vi "gugudan Client.vi"() -> ()   [LabVIEW 2014]
uses:
  <vilib>/Utility/sysdir.llb/System Directory Type.ctl
panel:
  out "email 2":string
  out "ip address":string=" ip address\r\n   서브넷 마스크 . . . . . . . : 255.255.255.0\r\n   기본 게이트웨이 . . . . . . : 192.168.0.1\r\n\r\n터널 어댑터 isatap.{E2E91750-802C-47E4-94E7-F6C5BD44A78B}:\r\n\r\n   미디어 상태 . . . . . . . . : 미디어 연결 끊김\r\n   연결별 DNS 접미사. . . . : \r\n\r\n터널 어댑터 로컬 영역 연결* 2:\r\n\r\n   연결별 DNS 접미사. . . . : \r\n   IPv6 주소 . . . . . . . . . : 2001:0:682f:9980:3c40:17a9:3f57:fff6\r\n   링크-로컬 IPv6 주소 . . . . : fe80::3c40:17a9:3f57:fff6%12\r\n   기본 게이트웨이 . . . . . . : ::\r\n"
  in  "제한해제":bool
  out "TIME":string="현재날자,시간"
  out "배열":string[][](array[string])
  out "email":string
  out "연결된 문자열":string
  out "abs(x)":i32
  out "문자열":string
  out "스페이스바3 2":string
  out "A  2":string
  out "D  2":string
  out "W 2":string
  out "W":string
  out "D":string
  out "A":string
  out "1":string
  out "2":string
  out "3":string
  out "스페이스바3":string
  out "key의숫자값":i16[](array[numeric])
  # "서비스를 이용해 주셔 감사합니다."
  # "서비스 종료를 위해서는 관리자 암호를 입력 해야 종료가 가능합니다."
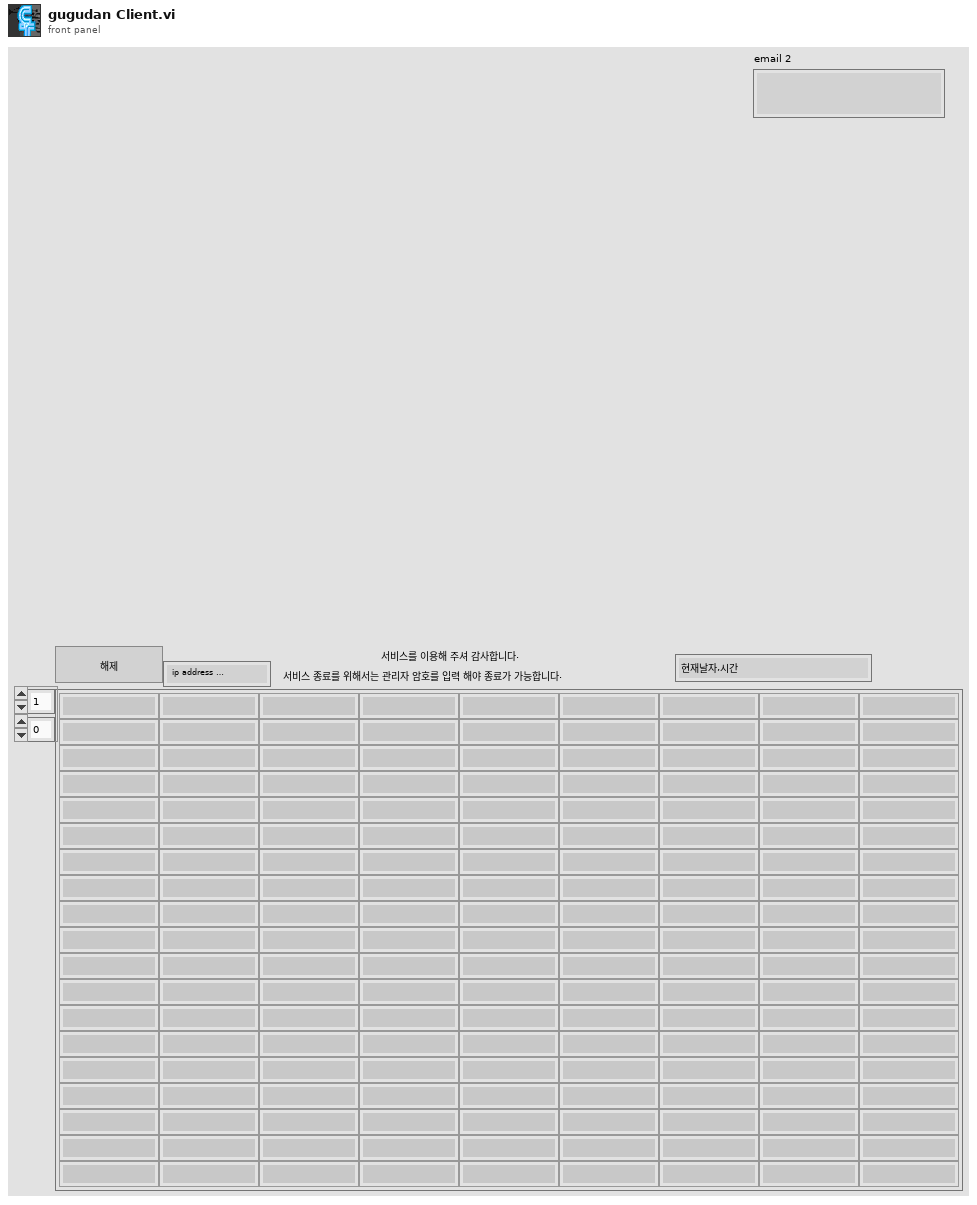
[diagram p1: front panel]
types:
  T1 = enum16{"open", "replace", "create", "open or create", "replace or create", "replace or create with confirmation"}
  T2 = typedef "System Directory Type.ctl" = i32
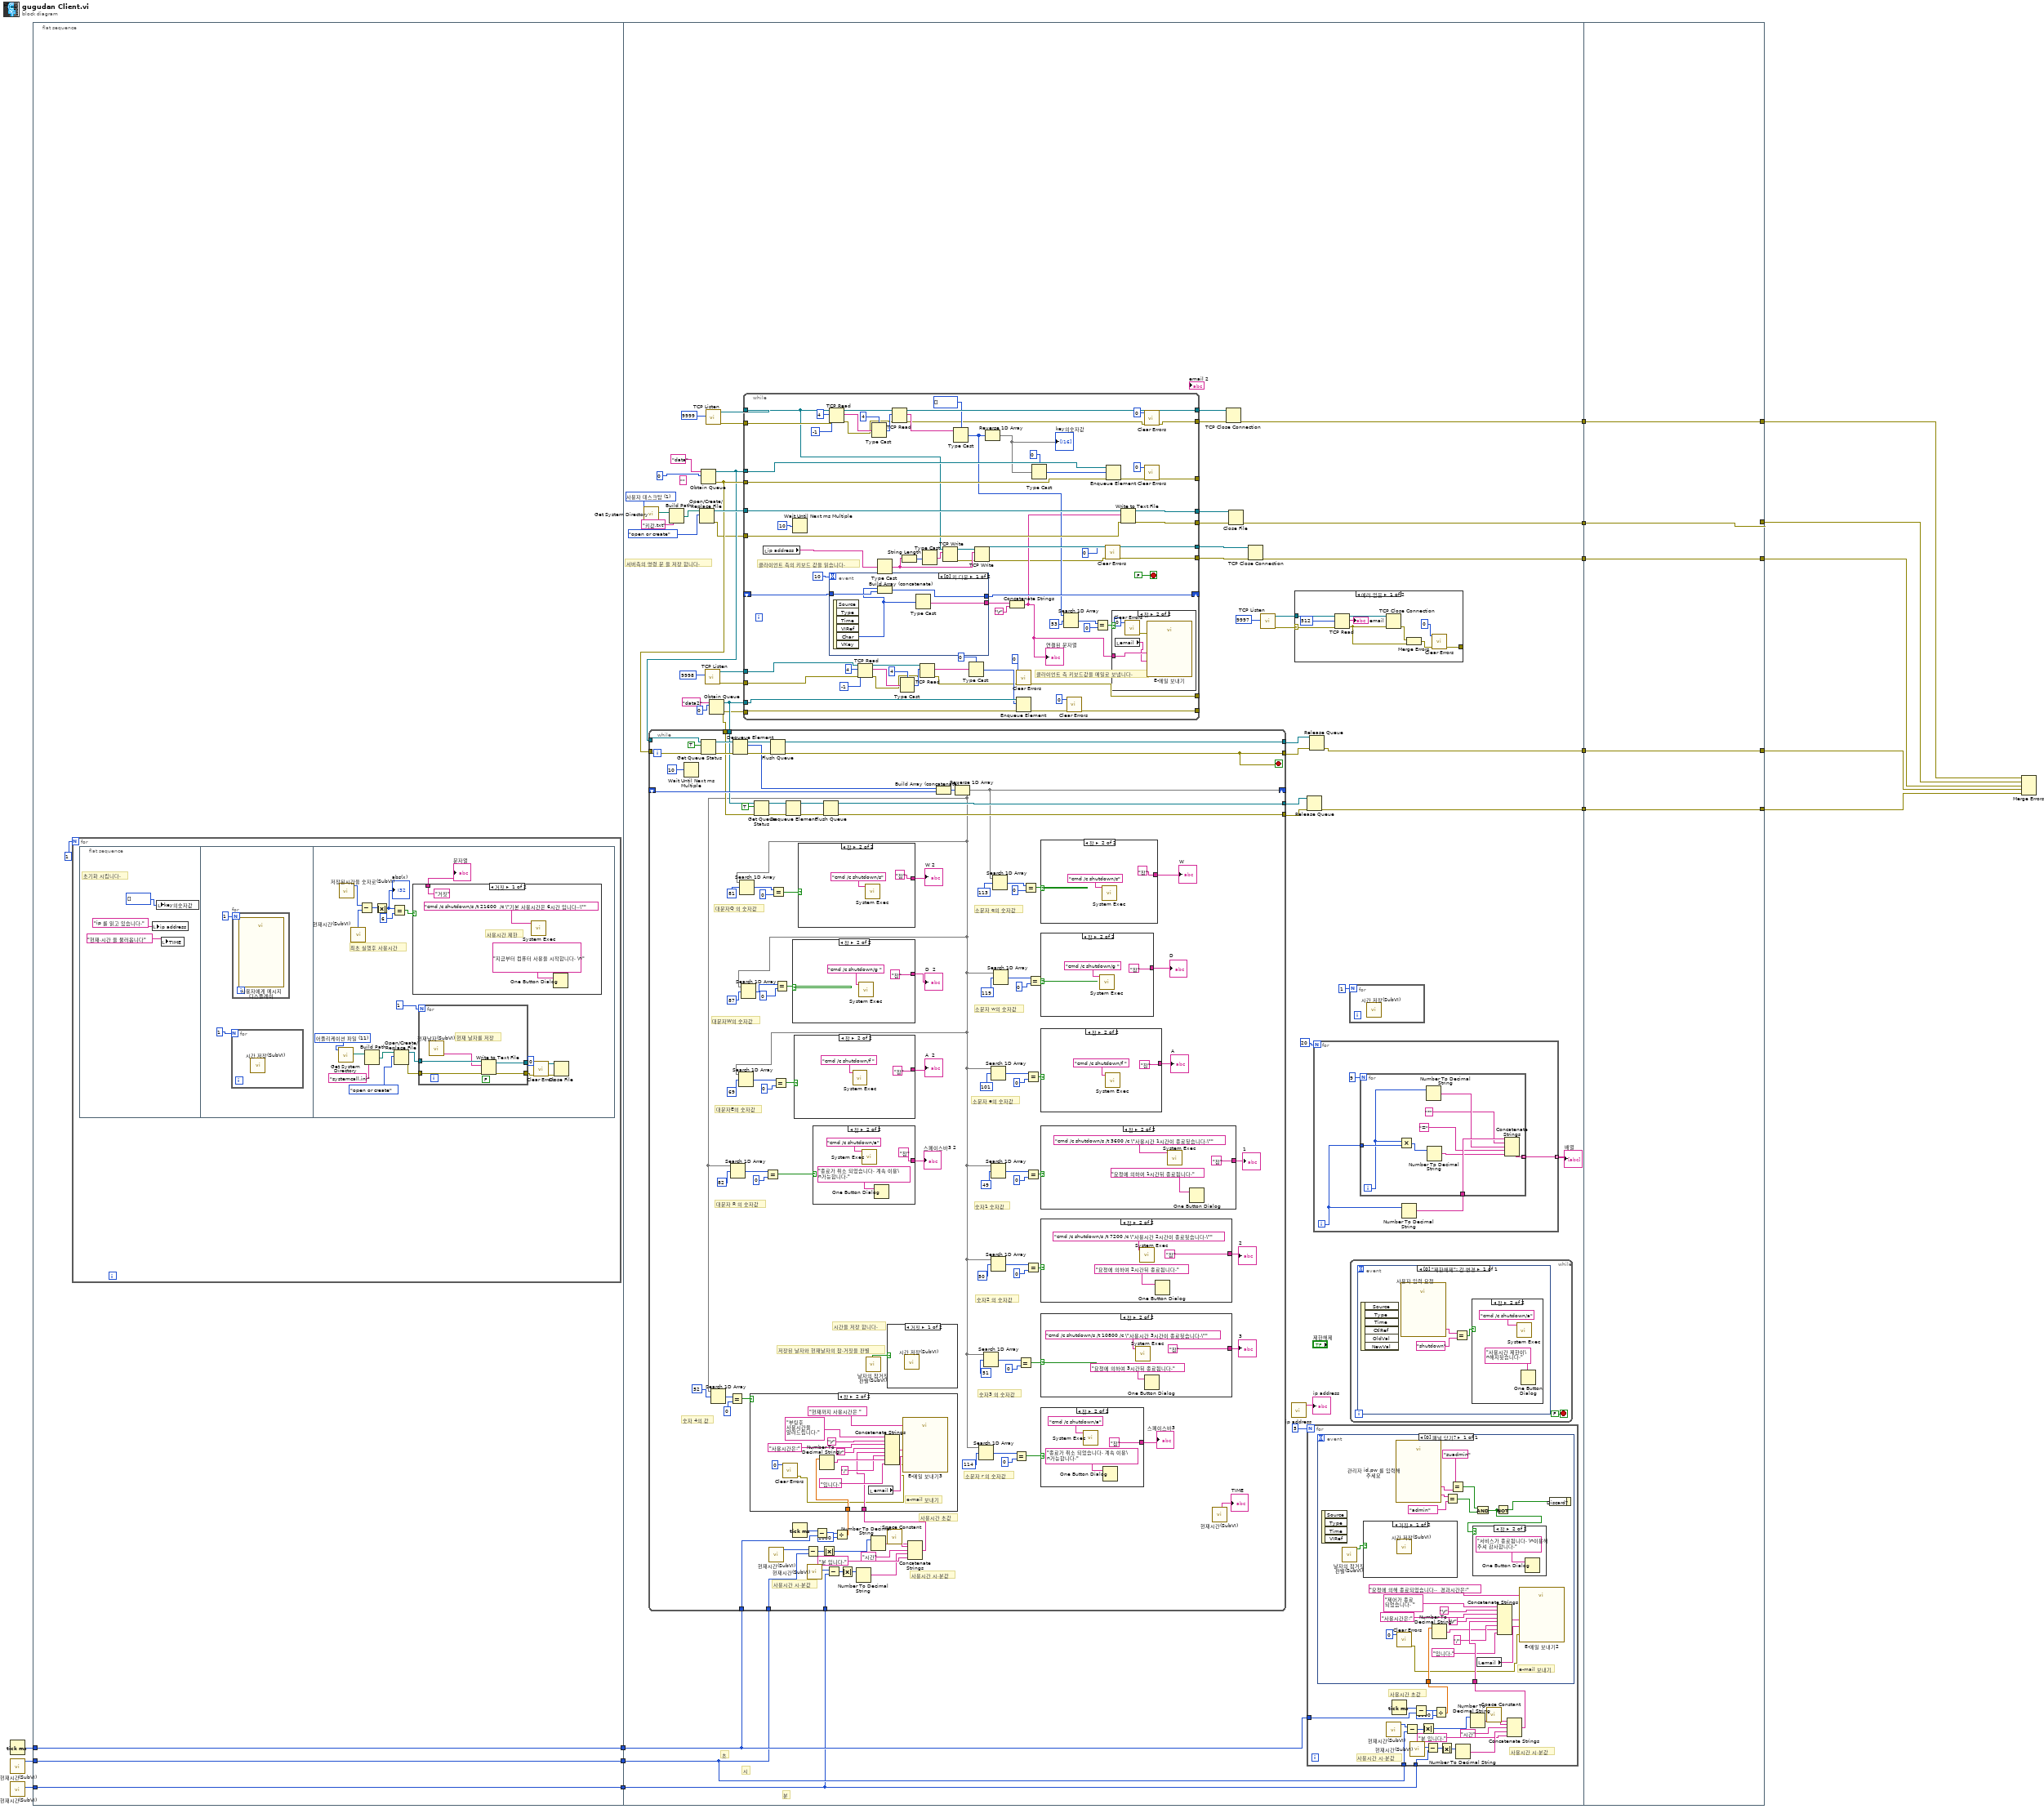
[diagram p0: block diagram]
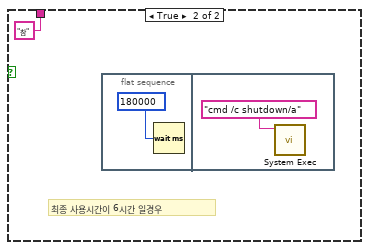
[diagram p2: hidden frame]
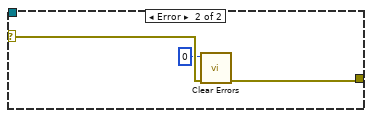
[diagram p4: hidden frame]
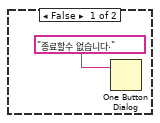
[diagram p6: hidden frame]
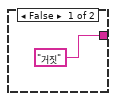
[diagram p9: hidden frame]
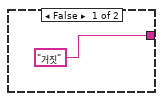
[diagram p10: hidden frame]
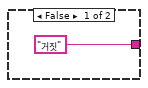
[diagram p11: hidden frame]
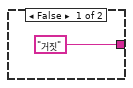
[diagram p12: hidden frame]
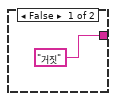
[diagram p13: hidden frame]
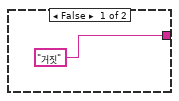
[diagram p14: hidden frame]
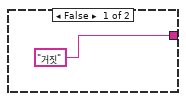
[diagram p15: hidden frame]
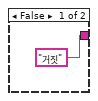
[diagram p16: hidden frame]
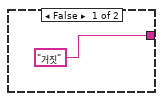
[diagram p17: hidden frame]
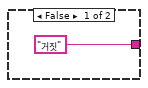
[diagram p18: hidden frame]
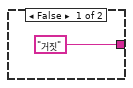
[diagram p19: hidden frame]
diagram:
  n1 = Tick Count (ms)() -> (millisecond timer value=w5:u32)
  n2 = call "현재시간(SubVI).vi"() -> ("시"=w4:i32)  [unwired: 3 in, 8 out]
  n3 = call "현재시간(SubVI).vi"() -> ("분"=w3:i32)  [unwired: 3 in, 8 out]
  n4 = flat-sequence {
    tunnel: [w19] -> w6
    tunnel: w5 -> [w19]
    tunnel: w4 -> [w18]
    tunnel: w3 -> [w17]
    tunnel: [w18] -> w2
    tunnel: [w17] -> w1
    tunnel: [w76] -> w16
    tunnel: [w67] -> w15
    tunnel: [w75] -> w14
    tunnel: [w74] -> w13
    tunnel: [w73] -> w12
    tunnel: w6 -> [w65]
    tunnel: w2 -> [w64]
    tunnel: w1 -> [w63]
    tunnel: w16 -> [w417]
    tunnel: w15 -> [w416]
    tunnel: w14 -> [w415]
    tunnel: w13 -> [w414]
    tunnel: w12 -> [w413]
    tunnel: [w417] -> w9
    tunnel: [w416] -> w8
    tunnel: [w415] -> w7
    tunnel: [w414] -> w10
    tunnel: [w413] -> w11
    frame #0 {
      n5 = for {
        N: 1 -> [_]
        n6 = flat-sequence {
          frame #0 {
            # "초기화 시킵니다."
            n7 = local write "ip address"("ip 를 읽고 있습니다.") -> ()
            n8 = local write "key의숫자값"(i16[] []) -> ()
            n9 = local write "TIME"("현재,시간 을 불러옵니다") -> ()
          }
          frame #1 {
            n10 = for {
              N: 1 -> [_]
              n11 = call "시간 저장(SubVI).vi"() -> ()  [unwired: 12 in]
            }
            n12 = for {
              N: 1 -> [_]
              n13 = call "사용자에게 메시지 디스플레이"() -> ()  [unwired: 10 in, 2 out]
            }
          }
          frame #2 {
            w28 = T2 11 items=["사용자 홈"=0, "사용자 데스크탑"=1, "사용자 문서"=2, "사용자 어플리케이션 데이터"=3, "사용자 환경"=4, "사용자 임시"=5, "퍼블릭 문서"=6, "퍼블릭 어플리케이션 데이터"=7, "퍼블릭 환경"=8, "퍼블릭 캐시"=13, "시스템 코어 라이브러리"=9, "시스템 설치된 라이브러리"=10, "어플리케이션 파일"=11, "부팅 볼륨 루트"=12] ("system directory type")
            # "최초 실행후 사용시간"
            n14 = call <vilib>:"Get System Directory.vi"("system directory type"=w28) -> ("system directory"=w33:path)  [unwired: 10 in]
            n15 = call "저장된시간을 숫자로(SubVI).vi"() -> ("저장된 문자를 숫자로"=w38:i32)  [unwired: 11 in]
            n16 = call "현재시간(SubVI).vi"() -> ("시"=w39:i32)  [unwired: 3 in, 8 out]
            n17 = Subtract(x=w38, y=w39) -> (x-y=w40:i32)
            n18 = Build Path(base path=w33, name or relative path="systemcall.ini" ("이름 또는 상대 경로")) -> (appended path=w31:path)
            n19 = Absolute Value(x=w40) -> (abs(x)=w42:i32)
            "abs(x)" <- w42
            n20 = Equal?(x=w42, y=6) -> (x = y?=w44:bool)
            n21 = Open/Create/Replace File(file path (use dialog)=w31, operation (0:open)=T1."open or create" ("동작(0:open)")) -> (refnum out=w29:refnum<file>, error out=w30:errorcluster)  [unwired: 4 in, 1 out]
            n22 = case shown="거짓" w44 {
              tunnel: ["거짓" "참"] -> w41
              frame False {
                # "사용시간 제한"
                n23 = call <vilib>:"System Exec.vi"("command line"="cmd /c shutdown/s /t 21600  /c \"기본 사용시간은 6시간 입니다..\"" ("standard input")) -> ()  [unwired: 7 in, 4 out]
                n24 = One Button Dialog(message="지금부터 컴퓨터 사용을 시작합니다. \n" ("메시지")) -> ()  [unwired: 1 in, 1 out]
              }
              frame True {
                # "최종 사용시간이 6시간 일경우"
                n25 = flat-sequence {
                  frame #0 {
                    n26 = Wait (ms)(milliseconds to wait=u32 180000 ("대기 시간(ms)")) -> ()  [unwired: 1 out]
                  }
                  frame #1 {
                    n27 = call <vilib>:"System Exec.vi"("command line"="cmd /c shutdown/a" ("standard input")) -> ()  [unwired: 7 in, 4 out]
                  }
                }
              }
            }
            "문자열" <- w41
            n28 = for {
              N: 1 -> [_]
              tunnel: w30 -> [w49]
              tunnel: [w48] -> w35
              tunnel: [w47] -> w34
              tunnel: w29 -> [w46]
              (unwired) FALSE
              # "현재 날자를 저장"
              n29 = call "현재날자(SubVI).vi"() -> ("월,일 을 문자열로"=w45:string)  [unwired: 5 in, 6 out]
              n30 = Write to Text File(file (use dialog)=w46, text=w45, error in=w49) -> (refnum out=w47:refnum<file>, error out=w48:errorcluster)  [unwired: 1 in, 1 out]
            }
            n31 = call <vilib>:"Clear Errors.vi"("error in (no error)"=w35, "specific error code to clear (0: all)"=0) -> ("error out"=w36:errorcluster)  [unwired: 4 in, 1 out]
            n32 = Close File(refnum=w34, error in=w36) -> ()  [unwired: 2 out]
          }
        }
      }
    }
    frame #1 {
      (unwired) ""
      w97 = T2 1 items=["사용자 홈"=0, "사용자 데스크탑"=1, "사용자 문서"=2, "사용자 어플리케이션 데이터"=3, "사용자 환경"=4, "사용자 임시"=5, "퍼블릭 문서"=6, "퍼블릭 어플리케이션 데이터"=7, "퍼블릭 환경"=8, "퍼블릭 캐시"=13, "시스템 코어 라이브러리"=9, "시스템 설치된 라이브러리"=10, "어플리케이션 파일"=11, "부팅 볼륨 루트"=12] ("system directory type")
      # "서버측의 명령 문 을 저장 합니다."
      # "초"
      # "분"
      # "시"
      n33 = call <vilib>:"Get System Directory.vi"("system directory type"=w97) -> ("system directory"=w96:path)  [unwired: 10 in]
      n34 = Build Path(base path=w96, name or relative path="키값.txt" ("이름 또는 상대 경로")) -> (appended path=w93:path)
      n35 = Open/Create/Replace File(file path (use dialog)=w93, operation (0:open)=T1."open or create" ("동작(0:open)")) -> (refnum out=w92:refnum<file>, error out=w71:errorcluster)  [unwired: 4 in, 1 out]
      n36 = Obtain Queue(name (unnamed)="data" ("이름(이름없음)"), element data type=i16 0) -> (queue out=w86:refnum<queue>, error out=w87:errorcluster)  [unwired: 3 in, 1 out]
      n37 = call <vilib>:"TCP Listen.vi"("port"=u16 9998) -> ("error out"=w83:errorcluster, "connection ID"=w84:refnum<k5>)  [unwired: 6 in, 3 out]
      n38 = call <vilib>:"TCP Listen.vi"("port"=u16 9999) -> ("error out"=w68:errorcluster, "connection ID"=w100:refnum<k5>)  [unwired: 6 in, 3 out]
      n39 = Obtain Queue(name (unnamed)="data2" ("이름(이름없음)"), element data type=i16 0) -> (queue out=w78:refnum<queue>, error out=w77:errorcluster)  [unwired: 3 in, 1 out]
      n40 = while {
        shift-right: [w180] -> _
        shift-left: _ -> [w245]
        tunnel: [w238] -> w89
        tunnel: [w237] -> w88
        tunnel: w86 -> [w244]
        tunnel: w87 -> [w243]
        tunnel: [w228] -> w80
        tunnel: [w227] -> w79
        tunnel: w78 -> [w206]
        tunnel: w77 -> [w205]
        tunnel: w65 -> [w185]
        tunnel: w64 -> [w184]
        tunnel: w63 -> [w183]
        stop <- w237 stop-if-true
        # "숫자 4의 값"
        # "저장된 날자와 현재날자의 참,거짓을 판별"
        # "시간을 저장 합니다."
        # "사용시간 시,분값"
        # "사용시간 시,분값"
        # "사용시간 초값"
        # "대문자 R 의 숫자값"
        # "대문자Q 의 숫자값"
        # "대문자W의 숫자값"
        # "대문자E의 숫자값"
        # "소문자 r 의 숫자값"
        # "숫자3 의 숫자값"
        # "소문자 q의 숫자값"
        # "소문자 w의 숫자값"
        # "소문자 e의 숫자값"
        # "숫자1 숫자값"
        # "숫자2 의 숫자값"
        n41 = Wait Until Next ms Multiple(millisecond multiple=u32 10) -> ()  [unwired: 1 out]
        n42 = Get Queue Status(queue=w244, return elements? (F)=TRUE ("원소 반환? (거짓)"), error in (no error)=w243) -> (queue out=w242:refnum<queue>, error out=w241:errorcluster)  [unwired: 6 out]
        n43 = Dequeue Element(queue=w242, error in (no error)=w241) -> (queue out=w239:refnum<queue>, element=w236:i16, error out=w240:errorcluster)  [unwired: 1 in, 1 out]
        n44 = Get Queue Status(queue=w206, return elements? (F)=TRUE ("원소 반환? (거짓)"), error in (no error)=w205) -> (queue out=w232:refnum<queue>, error out=w231:errorcluster)  [unwired: 6 out]
        n45 = call "현재시간(SubVI).vi"() -> ("시"=w187:i32)  [unwired: 3 in, 8 out]
        n46 = Flush Queue(queue=w239, error in (no error)=w240) -> (queue out=w238:refnum<queue>, error out=w237:errorcluster)  [unwired: 1 out]
        n47 = Dequeue Element(queue=w232, error in (no error)=w231) -> (queue out=w229:refnum<queue>, error out=w230:errorcluster)  [unwired: 1 in, 2 out]
        n48 = Tick Count (ms)() -> (millisecond timer value=w186:u32)
        n49 = Subtract(x=w187, y=w184) -> (x-y=w189:i32)
        n50 = call "현재시간(SubVI).vi"() -> ("분"=w188:i32)  [unwired: 3 in, 8 out]
        n51 = Subtract(x=w186, y=w185) -> (x-y=w198:u32)
        n52 = Absolute Value(x=w189) -> (abs(x)=w191:i32)
        n53 = Flush Queue(queue=w229, error in (no error)=w230) -> (queue out=w227:refnum<queue>, error out=w228:errorcluster)  [unwired: 1 out]
        n54 = Subtract(x=w188, y=w183) -> (x-y=w190:i32)
        n55 = Divide(x=w198, y=u32 1000) -> (x/y=w182:dbl)
        n56 = Absolute Value(x=w190) -> (abs(x)=w192:i32)
        n57 = Number To Decimal String(number=w192) -> (decimal integer string=w194:string)  [unwired: 1 in]
        n58 = call "날자의 참거짓 판별(SubVI).vi"() -> ("불리언"=w204:bool)  [unwired: 9 in, 2 out]
        n59 = Number To Decimal String(number=w191) -> (decimal integer string=w196:string)  [unwired: 1 in]
        n60 = call <vilib>:"Space Constant.vi"() -> ("String"=w197:string)
        n61 = case shown="거짓" w204 {
          frame False {
            n62 = call "시간 저장(SubVI).vi"() -> ()  [unwired: 12 in]
          }
          frame True {
          }
        }
        n63 = Concatenate Strings(w196, w197, "시간", w194, "분 입니다.") -> (w181:string)
        n64 = Build Array (concatenate)(w236, w245) -> (w234:i16[])
        n65 = Reverse 1D Array(array=w234) -> (reversed array=w180:i16[])
        n66 = Search 1D Array(1D array=w180, element=i16 52 ("원소")) -> (index of element=w202:i32)  [unwired: 1 in]
        n67 = Equal?(x=w202, y=0) -> (x = y?=w200:bool)
        n68 = Search 1D Array(1D array=w180, element=i16 82 ("원소")) -> (index of element=w209:i32)  [unwired: 1 in]
        n69 = Search 1D Array(1D array=w180, element=i16 69 ("원소")) -> (index of element=w214:i32)  [unwired: 1 in]
        n70 = Search 1D Array(1D array=w180, element=i16 81 ("원소")) -> (index of element=w224:i32)  [unwired: 1 in]
        n71 = Search 1D Array(1D array=w180, element=i16 87 ("원소")) -> (index of element=w222:i32)  [unwired: 1 in]
        n72 = case shown="참" w200 {
          tunnel: w182 -> [_ w286]
          tunnel: w181 -> [_ w285]
          frame False {
          }
          frame True {
            # "e-mail 보내기"
            n73 = call <vilib>:"Clear Errors.vi"("specific error code to clear (0: all)"=0) -> ("error out"=w282:errorcluster)  [unwired: 5 in, 1 out]
            n74 = Number To Decimal String(number=w286) -> (decimal integer string=w294:string)  [unwired: 1 in]
            n75 = local read "email"() -> (w284:string)
            n76 = Concatenate Strings("부팅후 사용시간을 알려드립니다." ("문자열"), "\r", "사용시간은:", "\r", w285, "/", w294, "입니다.") -> (w291:string)
            n77 = call "E-메일 보내기3"("error in"=w282, "Message"=w291, "Subject"="현재까지 사용시간은 ", "Recipients"=w284) -> ()  [unwired: 7 in, 1 out]
          }
        }
        n78 = Equal?(x=w209, y=0) -> (x = y?=w211:bool)
        n79 = Equal?(x=w224, y=0) -> (x = y?=w221:bool)
        n80 = Equal?(x=w214, y=0) -> (x = y?=w216:bool)
        n81 = Equal?(x=w222, y=0) -> (x = y?=w219:bool)
        n82 = case shown="참" w219 {
          tunnel: ["거짓" "참"] -> w220
          frame False {
          }
          frame True {
            n83 = call <vilib>:"System Exec.vi"("command line"="cmd /c shutdown/g " ("standard input")) -> ()  [unwired: 7 in, 4 out]
          }
        }
        "D  2" <- w220
        n84 = case shown="참" w216 {
          tunnel: ["거짓" "참"] -> w215
          frame False {
          }
          frame True {
            n85 = call <vilib>:"System Exec.vi"("command line"="cmd /c shutdown/f " ("standard input")) -> ()  [unwired: 7 in, 4 out]
          }
        }
        "A  2" <- w215
        n86 = case shown="참" w221 {
          tunnel: ["거짓" "참"] -> w226
          frame False {
          }
          frame True {
            n87 = call <vilib>:"System Exec.vi"("command line"="cmd /c shutdown/s" ("standard input")) -> ()  [unwired: 7 in, 4 out]
          }
        }
        "W 2" <- w226
        n88 = case shown="참" w211 {
          tunnel: ["거짓" "참"] -> w207
          frame False {
          }
          frame True {
            n89 = call <vilib>:"System Exec.vi"("command line"="cmd /c shutdown/a" ("standard input")) -> ()  [unwired: 7 in, 4 out]
            n90 = One Button Dialog(message="종료가 취소 되었습니다. 계속 이용\n가능합니다." ("메시지")) -> ()  [unwired: 1 in, 1 out]
          }
        }
        "스페이스바3 2" <- w207
        n91 = Search 1D Array(1D array=w180, element=i16 114 ("원소")) -> (index of element=w250:i32)  [unwired: 1 in]
        n92 = Search 1D Array(1D array=w180, element=i16 51 ("원소")) -> (index of element=w255:i32)  [unwired: 1 in]
        n93 = Search 1D Array(1D array=w180, element=i16 101 ("원소")) -> (index of element=w269:i32)  [unwired: 1 in]
        n94 = Search 1D Array(1D array=w180, element=i16 49 ("원소")) -> (index of element=w268:i32)  [unwired: 1 in]
        n95 = Search 1D Array(1D array=w180, element=i16 50 ("원소")) -> (index of element=w261:i32)  [unwired: 1 in]
        n96 = Search 1D Array(1D array=w180, element=i16 113 ("원소")) -> (index of element=w279:i32)  [unwired: 1 in]
        n97 = Search 1D Array(1D array=w180, element=i16 119 ("원소")) -> (index of element=w277:i32)  [unwired: 1 in]
        n98 = Equal?(x=w250, y=0) -> (x = y?=w252:bool)
        n99 = Equal?(x=w255, y=0) -> (x = y?=w253:bool)
        n100 = Equal?(x=w279, y=0) -> (x = y?=w276:bool)
        n101 = Equal?(x=w269, y=0) -> (x = y?=w271:bool)
        n102 = Equal?(x=w268, y=0) -> (x = y?=w266:bool)
        n103 = Equal?(x=w261, y=0) -> (x = y?=w263:bool)
        n104 = Equal?(x=w277, y=0) -> (x = y?=w274:bool)
        n105 = case shown="참" w276 {
          tunnel: ["거짓" "참"] -> w281
          frame False {
          }
          frame True {
            n106 = call <vilib>:"System Exec.vi"("command line"="cmd /c shutdown/s" ("standard input")) -> ()  [unwired: 7 in, 4 out]
          }
        }
        "W" <- w281
        n107 = case shown="참" w274 {
          tunnel: ["거짓" "참"] -> w275
          frame False {
          }
          frame True {
            n108 = call <vilib>:"System Exec.vi"("command line"="cmd /c shutdown/g " ("standard input")) -> ()  [unwired: 7 in, 4 out]
          }
        }
        "D" <- w275
        n109 = case shown="참" w271 {
          tunnel: ["거짓" "참"] -> w270
          frame False {
          }
          frame True {
            n110 = call <vilib>:"System Exec.vi"("command line"="cmd /c shutdown/f " ("standard input")) -> ()  [unwired: 7 in, 4 out]
          }
        }
        "A" <- w270
        n111 = case shown="참" w266 {
          tunnel: ["거짓" "참"] -> w267
          frame False {
          }
          frame True {
            n112 = call <vilib>:"System Exec.vi"("command line"="cmd /c shutdown/s /t 3600 /c \"사용시간 1시간이 종료됫습니다.\"" ("standard input")) -> ()  [unwired: 7 in, 4 out]
            n113 = One Button Dialog(message="요청에 의하여 1시간뒤 종료됩니다." ("메시지")) -> ()  [unwired: 1 in, 1 out]
          }
        }
        "1" <- w267
        n114 = case shown="참" w263 {
          tunnel: ["거짓" "참"] -> w262
          frame False {
          }
          frame True {
            n115 = call <vilib>:"System Exec.vi"("command line"="cmd /c shutdown/s /t 7200 /c \"사용시간 2시간이 종료됫습니다.\"" ("standard input")) -> ()  [unwired: 7 in, 4 out]
            n116 = One Button Dialog(message="요청에 의하여 2시간뒤 종료됩니다." ("메시지")) -> ()  [unwired: 1 in, 1 out]
          }
        }
        "2" <- w262
        n117 = case shown="참" w253 {
          tunnel: ["거짓" "참"] -> w235
          frame False {
          }
          frame True {
            n118 = call <vilib>:"System Exec.vi"("command line"="cmd /c shutdown/s /t 10800 /c \"사용시간 3시간이 종료됫습니다.\"" ("standard input")) -> ()  [unwired: 7 in, 4 out]
            n119 = One Button Dialog(message="요청에 의하여 3시간뒤 종료됩니다." ("메시지")) -> ()  [unwired: 1 in, 1 out]
          }
        }
        "3" <- w235
        n120 = case shown="참" w252 {
          tunnel: ["거짓" "참"] -> w248
          frame False {
          }
          frame True {
            n121 = call <vilib>:"System Exec.vi"("command line"="cmd /c shutdown/a" ("standard input")) -> ()  [unwired: 7 in, 4 out]
            n122 = One Button Dialog(message="종료가 취소 되었습니다. 계속 이용\n가능합니다." ("메시지")) -> ()  [unwired: 1 in, 1 out]
          }
        }
        "스페이스바3" <- w248
        n123 = call "현재시간(SubVI).vi"() -> ("날짜/시간 문자열"=→"TIME":string)  [unwired: 3 in, 8 out]
      }
      n124 = while {
        tunnel: w100 -> [w334]
        tunnel: [w403] -> w101
        tunnel: [w396] -> w99
        tunnel: w92 -> [w389]
        tunnel: [w390] -> w98
        tunnel: w86 -> [w388]
        tunnel: w87 -> [w387]
        shift-right: [w379] -> _
        shift-left: _ -> [w380]
        tunnel: w84 -> [w335]
        tunnel: w83 -> [w371]
        tunnel: w78 -> [w366]
        tunnel: w77 -> [w367]
        tunnel: [w339] -> w72
        tunnel: w71 -> [w363]
        tunnel: [w362] -> w70
        tunnel: [w351] -> w69
        tunnel: w68 -> [w360]
        tunnel: [w348] -> _
        tunnel: [w344] -> _
        tunnel: [w341] -> _
        stop <- FALSE stop-if-true
        # "클라이언트 측 키보드값을 메일로 보냅니다."
        # "클라이언트 측의 키보드 값을 읽습니다."
        n125 = local read "ip address"() -> (w336:string)
        n126 = Wait Until Next ms Multiple(millisecond multiple=u32 10) -> ()  [unwired: 1 out]
        n127 = TCP Read(connection ID=w334, bytes to read=4, error in (no error)=w360, 9:-1 ("타임아웃 ms (25000)")) -> (connection ID out=w393:refnum<k5>, data out=w395:string, error out=w361:errorcluster)  [unwired: 1 in]
        n128 = event shown="[0] 키 다운" {
          selector: _ -> [_ _]
          dyn-events: _ -> [_ _]
          timeout: 10 -> [_ _]
          tunnel: [w410 w412] -> w379
          tunnel: w380 -> [w411 w412]
          tunnel: [w408 _] -> w359
          event Key Down {
            n129 = event-data() -> ("Char"=w409:i16)  [unwired: 1 in, 5 out]
            n130 = Build Array (concatenate)(w409, w411) -> (w410:i16[])
            n131 = Type Cast(x=w409) -> (*(type *) &x=w408:string)  [unwired: 1 in]
          }
          event Timeout {
            n132 = event-data() -> ()  [unwired: 1 in, 3 out]
          }
        }
        n133 = TCP Read(connection ID=w335, bytes to read=4, error in (no error)=w371, 9:-1 ("타임아웃 ms (25000)")) -> (connection ID out=w374:refnum<k5>, data out=w372:string, error out=w370:errorcluster)  [unwired: 1 in]
        n134 = Type Cast(type=4 ("bytes to read"), x=w395) -> (*(type *) &x=w385:i32)
        n135 = Type Cast(x=w336) -> (*(type *) &x=w397:string)  [unwired: 1 in]
        n136 = TCP Read(connection ID=w393, bytes to read=w385, error in (no error)=w361) -> (connection ID out=w403:refnum<k5>, data out=w386:string, error out=w350:errorcluster)  [unwired: 2 in]
        n137 = Type Cast(type=4 ("bytes to read"), x=w372) -> (*(type *) &x=w377:i32)
        n138 = String Length(string=w397) -> (length=w398:i32)
        n139 = TCP Read(connection ID=w374, bytes to read=w377, error in (no error)=w370) -> (data out=w369:string, error out=w342:errorcluster)  [unwired: 2 in, 1 out]
        n140 = Type Cast(x=w398) -> (*(type *) &x=w399:string)  [unwired: 1 in]
        n141 = TCP Write(connection ID=w334, data in=w399) -> (connection ID out=w400:refnum<k5>, error out=w364:errorcluster)  [unwired: 2 in, 1 out]
        n142 = Type Cast(type=i16[] [], x=w386) -> (*(type *) &x=w354:i16[])
        n143 = Type Cast(type=i16 0, x=w369) -> (*(type *) &x=w365:i16)
        n144 = TCP Write(connection ID=w400, data in=w397, error in (no error)=w364) -> (connection ID out=w396:refnum<k5>, error out=w338:errorcluster)  [unwired: 1 in, 1 out]
        n145 = Reverse 1D Array(array=w354) -> (reversed array=w381:i16[])
        "key의숫자값" <- w381
        n146 = Concatenate Strings(w359, "\r") -> (w352:string)
        "연결된 문자열" <- w352
        n147 = Enqueue Element(queue=w366, element=w365, error in (no error)=w367) -> (error out=w345:errorcluster)  [unwired: 1 in, 2 out]
        n148 = call <vilib>:"Clear Errors.vi"("error in (no error)"=w342, "specific error code to clear (0: all)"=0) -> ("error out"=w341:errorcluster)  [unwired: 4 in, 1 out]
        n149 = Type Cast(type=i16 0, x=w381) -> (*(type *) &x=w383:i16)
        n150 = Search 1D Array(1D array=w354, element=i16 53 ("원소")) -> (index of element=w357:i32)  [unwired: 1 in]
        n151 = call <vilib>:"Clear Errors.vi"("error in (no error)"=w345, "specific error code to clear (0: all)"=0) -> ("error out"=w344:errorcluster)  [unwired: 4 in, 1 out]
        n152 = Equal?(x=w357, y=0) -> (x = y?=w353:bool)
        n153 = call <vilib>:"Clear Errors.vi"("error in (no error)"=w338, "specific error code to clear (0: all)"=0) -> ("error out"=w339:errorcluster)  [unwired: 4 in, 1 out]
        n154 = Enqueue Element(queue=w388, element=w383, error in (no error)=w387) -> (error out=w349:errorcluster)  [unwired: 1 in, 2 out]
        n155 = case shown="참" w353 {
          tunnel: w352 -> [_ w407]
          frame False {
          }
          frame True {
            n156 = local read "email"() -> (w406:string)
            n157 = call <vilib>:"Clear Errors.vi"("specific error code to clear (0: all)"=0) -> ("error out"=w404:errorcluster)  [unwired: 5 in, 1 out]
            n158 = call "E-메일 보내기"("error in"=w404, "Message"=w407, "Recipients"=w406) -> ()  [unwired: 8 in, 1 out]
          }
        }
        n159 = Write to Text File(file (use dialog)=w389, text=w352, error in=w363) -> (refnum out=w390:refnum<file>, error out=w362:errorcluster)  [unwired: 1 in, 1 out]
        n160 = call <vilib>:"Clear Errors.vi"("error in (no error)"=w350, "specific error code to clear (0: all)"=0) -> ("error out"=w351:errorcluster)  [unwired: 4 in, 1 out]
        n161 = call <vilib>:"Clear Errors.vi"("error in (no error)"=w349, "specific error code to clear (0: all)"=0) -> ("error out"=w348:errorcluster)  [unwired: 4 in, 1 out]
      }
      n162 = TCP Close Connection(connection ID=w101, error in (no error)=w69) -> (error out=w73:errorcluster)  [unwired: 1 in, 1 out]
      n163 = Close File(refnum=w98, error in=w70) -> (error out=w74:errorcluster)  [unwired: 1 out]
      n164 = TCP Close Connection(connection ID=w99, error in (no error)=w72) -> (error out=w75:errorcluster)  [unwired: 1 in, 1 out]
      n165 = call <vilib>:"TCP Listen.vi"("port"=u16 9997) -> ("error out"=w60:errorcluster, "connection ID"=w61:refnum<k5>)  [unwired: 6 in, 3 out]
      n166 = call "ip address.vi"() -> ("ip address"=→"ip address":string)  [unwired: 11 in]
      n167 = case shown="에러 없음" w60 {
        selector: w60 -> [w127 w133]
        tunnel: [w124 w134] -> _
        tunnel: w61 -> [w131 _]
        frame No Error {
          n168 = TCP Read(connection ID=w131, bytes to read=512, error in (no error)=w127) -> (connection ID out=w126:refnum<k5>, data out=→"email":string, error out=w125:errorcluster)  [unwired: 2 out]
          n169 = TCP Close Connection(connection ID=w126, error in (no error)=w125) -> (error out=w128:errorcluster)  [unwired: 2 out]
          n170 = Merge Errors(w128, w125) -> (w123:errorcluster)
          n171 = call <vilib>:"Clear Errors.vi"("error in (no error)"=w123, "specific error code to clear (0: all)"=0) -> ("error out"=w124:errorcluster)  [unwired: 4 in, 1 out]
        }
        frame Error {
          n172 = call <vilib>:"Clear Errors.vi"("error in (no error)"=w133, "specific error code to clear (0: all)"=0) -> ("error out"=w134:errorcluster)  [unwired: 4 in, 1 out]
        }
      }
      n173 = Release Queue(queue=w79, error in (no error)=w80) -> (error out=w67:errorcluster)  [unwired: 1 in, 2 out]
      n174 = for {
        N: 5 -> [_]
        tunnel: w65 -> [w152]
        tunnel: w64 -> [w150]
        tunnel: w63 -> [w148]
        # "사용시간 시,분값"
        # "사용시간 시,분값"
        # "사용시간 초값"
        n175 = call "현재시간(SubVI).vi"() -> ("시"=w151:i32)  [unwired: 3 in, 8 out]
        n176 = Tick Count (ms)() -> (millisecond timer value=w153:u32)
        n177 = Subtract(x=w151, y=w150) -> (x-y=w147:i32)
        n178 = call "현재시간(SubVI).vi"() -> ("분"=w149:i32)  [unwired: 3 in, 8 out]
        n179 = Subtract(x=w153, y=w152) -> (x-y=w138:u32)
        n180 = Absolute Value(x=w147) -> (abs(x)=w145:i32)
        n181 = Subtract(x=w149, y=w148) -> (x-y=w146:i32)
        n182 = Divide(x=w138, y=u32 1000) -> (x/y=w136:dbl)
        n183 = Absolute Value(x=w146) -> (abs(x)=w144:i32)
        n184 = Number To Decimal String(number=w144) -> (decimal integer string=w142:string)  [unwired: 1 in]
        n185 = Number To Decimal String(number=w145) -> (decimal integer string=w140:string)  [unwired: 1 in]
        n186 = call <vilib>:"Space Constant.vi"() -> ("String"=w139:string)
        n187 = Concatenate Strings(w140, w139, "시간", w142, "분 입니다.") -> (w135:string)
        n188 = event shown="[0] 패널 닫기?" {
          selector: _ -> [_]
          dyn-events: _ -> [_]
          timeout: _ -> [_]
          tunnel: w136 -> [w168]
          tunnel: w135 -> [w161]
          event Panel Close? {
            # "e-mail 보내기"
            n189 = event-data() -> ()  [unwired: 1 in, 4 out]
            n190 = call "날자의 참거짓 판별(SubVI).vi"() -> ("불리언"=w157:bool)  [unwired: 9 in, 2 out]
            n191 = case shown="거짓" w157 {
              frame False {
                n192 = call "시간 저장(SubVI).vi"() -> ()  [unwired: 12 in]
              }
              frame True {
              }
            }
            n193 = call "관리자 id.pw 를 입력해 주세요"() -> ("PW"=w176:string, "ID"=w173:string)  [unwired: 16 in, 2 out]
            n194 = call <vilib>:"Clear Errors.vi"("specific error code to clear (0: all)"=0) -> ("error out"=w155:errorcluster)  [unwired: 5 in, 1 out]
            n195 = Number To Decimal String(number=w168) -> (decimal integer string=w159:string)  [unwired: 1 in]
            n196 = Equal?(x=w176, y="admin") -> (x = y?=w172:bool)
            n197 = Equal?(x="suadmin", y=w173) -> (x = y?=w171:bool)
            n198 = And(x=w171, y=w172) -> (x .and. y?=w169:bool)
            n199 = case shown="참" w169 {
              frame False {
                n200 = One Button Dialog(message="종료할수 없습니다." ("메시지")) -> ()  [unwired: 1 in, 1 out]
              }
              frame True {
                n201 = One Button Dialog(message="서비스가 종료됩니다. \n이용해 주셔 감사합니다." ("메시지")) -> ()  [unwired: 1 in, 1 out]
              }
            }
            n202 = local read "email"() -> (w156:string)
            n203 = Not(x=w169) -> (.not. x?=w170:bool)
            n204 = Concatenate Strings("제어가 종료 되었습니다. " ("문자열"), "\r", "사용시간은:", "\r", w161, "/", w159, "입니다.") -> (w163:string)
            n205 = call "E-메일 보내기2"("error in"=w155, "Message"=w163, "Subject"="요청에 의해 종료되었습니다,.  경과시간은:", "Recipients"=w156) -> ()  [unwired: 7 in, 1 out]
            n206 = event-data("Discard?"=w170) -> ()  [unwired: 1 in, 1 out]
          }
        }
      }
      n207 = Release Queue(queue=w89, error in (no error)=w88) -> (error out=w76:errorcluster)  [unwired: 1 in, 2 out]
      n208 = for {
        N: 20 -> [_]
        tunnel: [w109] -> w58 mode=indexing
        i -> [w111]
        n209 = Number To Decimal String(number=w111) -> (decimal integer string=w110:string)  [unwired: 1 in]
        n210 = for {
          N: 9 -> [_]
          tunnel: w111 -> [w121]
          tunnel: w110 -> [w119]
          tunnel: [w114] -> w109 mode=indexing
          i -> [w113]
          n211 = Multiply(x=w113, y=w121) -> (x*y=w120:i32)
          n212 = Number To Decimal String(number=w113) -> (decimal integer string=w118:string)  [unwired: 1 in]
          n213 = Number To Decimal String(number=w120) -> (decimal integer string=w115:string)  [unwired: 1 in]
          n214 = Concatenate Strings(w119, "*", w118, "=", w115) -> (w114:string)
        }
      }
      "배열" <- w58
      n215 = for {
        N: 1 -> [_]
        n216 = call "시간 저장(SubVI).vi"() -> ()  [unwired: 12 in]
      }
      n217 = while {
        stop <- FALSE stop-if-true
        n218 = event shown="[0] \"제한해제\": 값 변경" {
          selector: _ -> [_]
          dyn-events: _ -> [_]
          timeout: _ -> [_]
          event "제한해제": Value Change {
            n219 = event-data() -> ()  [unwired: 1 in, 6 out]
            n220 = call "사용자 입력 요청"() -> ("종료 취소"=w105:string)  [unwired: 17 in, 2 out]
            n221 = Equal?(x=w105, y="shutdown") -> (x = y?=w104:bool)
            n222 = case shown="참" w104 {
              frame False {
              }
              frame True {
                n223 = call <vilib>:"System Exec.vi"("command line"="cmd /c shutdown/a" ("standard input")) -> ()  [unwired: 7 in, 4 out]
                n224 = One Button Dialog(message="사용시간 제한이\n해지됫습니다." ("메시지")) -> ()  [unwired: 1 in, 1 out]
              }
            }
          }
        }
      }
    }
    frame #2 {
    }
  }
  n225 = Merge Errors(w11, w10, w7, w9, w8) -> ()  [unwired: 1 out]
